vi "SH_ComputeThreshold.vi"(4 "Shapelet Length":i32, 5 "ShapeletClass in":refnum<class "Shapelets Search Brute Force.lvclass">) -> (0 "percentile":dbl, 2 "ShapeletClass out":refnum<class "Shapelets Search Brute Force.lvclass">)   [LabVIEW 2016, in "Shapelets Search (Brute Force).lvlib" / "Shapelets Search Brute Force.lvclass"]
uses:
  Shapelets Search Brute Force.lvclass
  Shapelets Search Brute Force.lvclass/Shapelets Search Brute Force.ctl
  <vilib>/Analysis/baseanly.llb/Normalize Vector.vi
  <vilib>/gmath/statdist.llb/Uniform (Discrete) Random.vi
  <vilib>/gmath/statdist.llb/st_Percentiles (scalar).vi
  <vilib>/gmath/NI_Gmath.lvlib
  <vilib>/Analysis/NI_AALBase.lvlib
panel:
  # "This VI is a part of BCI Design library, http://www.ru-bci.org \nCopyright © 2020, Sotnikov Peter, All rights reserved. License: GNU GPLv3"
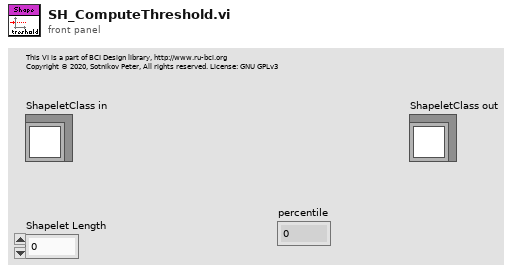
[diagram p1: front panel]
types:
  T1 = cluster{"ClassLabel":string, "FeatureVector":dbl[][]}[]
  T2 = cluster{"ClassLabel":string, "FeatureVector":dbl[][]}
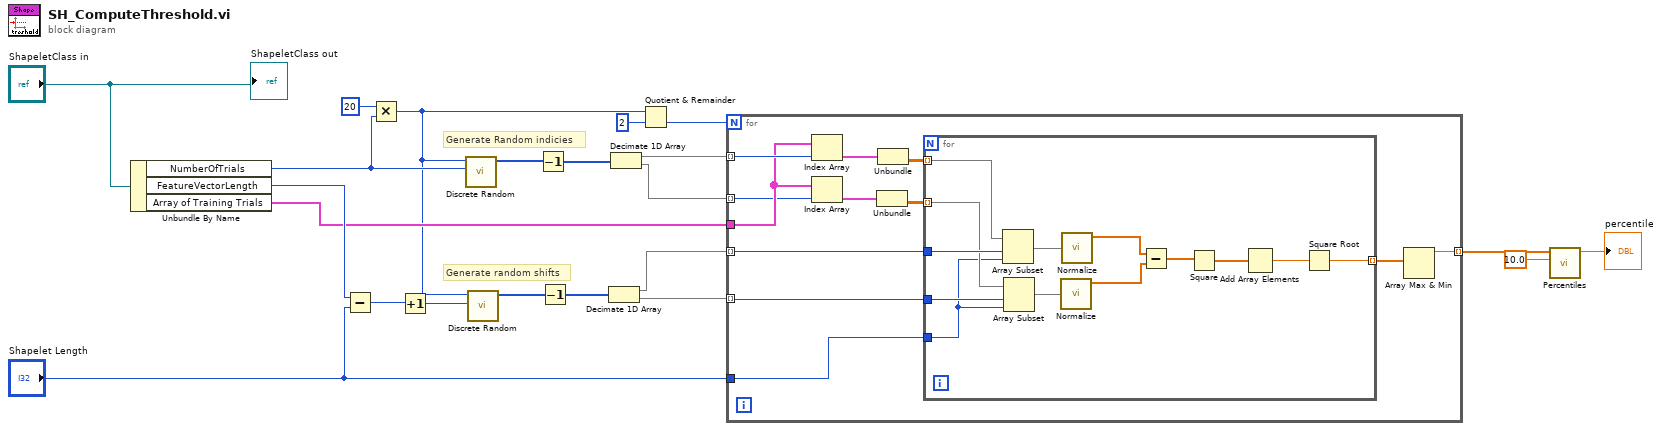
[diagram p0: block diagram]
diagram:
  # "Generate Random indicies"
  # "Generate random shifts"
  n1 = Unbundle By Name("ShapeletClass in") -> ("NumberOfTrials"=w6:i32, "FeatureVectorLength"=w21:i32, "Array of Training Trials"=w14:T1)
  n2 = Subtract(x=w21, y="Shapelet Length") -> (x-y=w8:i32)
  n3 = Multiply(x=20, y=w6) -> (x*y=w5:i32)
  n4 = Increment(x=w8) -> (x+1=w7:i32)
  n5 = call-poly <vilib>:"Discrete Random.vi"("n"=w6, "samples"=w5) -> ("uniform (discrete) random data"=w12:i32[])  [unwired: 8 in, 1 out]
  n6 = call-poly <vilib>:"Discrete Random.vi"("n"=w7, "samples"=w5) -> ("uniform (discrete) random data"=w10:i32[])  [unwired: 8 in, 1 out]
  n7 = Decrement(x=w12) -> (x-1=w11:i32[])
  n8 = Decrement(x=w10) -> (x-1=w9:i32[])
  n9 = Decimate 1D Array(w9) -> (w16:i32[], w15:i32[])
  n10 = Decimate 1D Array(w11) -> (w18:i32[], w17:i32[])
  n11 = Quotient & Remainder(x=w5, y=2) -> (floor(x/y)=w19:i32)  [unwired: 1 out]
  n12 = for {
    N: w19 -> [_]
    tunnel: w18 -> [w34] mode=indexing
    tunnel: w17 -> [w32] mode=indexing
    tunnel: w16 -> [w29] mode=indexing
    tunnel: w15 -> [w28] mode=indexing
    tunnel: w14 -> [w33]
    tunnel: "Shapelet Length" -> [w25]
    tunnel: [w23] -> w3 mode=indexing
    n13 = Index Array(array=w33, index=w34) -> (element=w31:T2)
    n14 = Index Array(array=w33, index=w32) -> (element=w30:T2)
    n15 = Unbundle(w30) -> ("FeatureVector"=w26:dbl[][])  [unwired: 1 out]
    n16 = Unbundle(w31) -> ("FeatureVector"=w27:dbl[][])  [unwired: 1 out]
    n17 = for {
      tunnel: w29 -> [w47]
      tunnel: w28 -> [w46]
      tunnel: w27 -> [w45] mode=indexing
      tunnel: w26 -> [w44] mode=indexing
      tunnel: w25 -> [w37]
      tunnel: [w36] -> w24 mode=indexing
      n18 = Array Subset(array=w45, index=w47, length=w37) -> (w43:dbl[])
      n19 = Array Subset(array=w44, index=w46, length=w37) -> (w42:dbl[])
      n20 = call-poly <vilib>:"Normalize.vi"("Vector"=w42) -> ("Normalized Vector"=w40:dbl[])  [unwired: 1 in, 3 out]
      n21 = call-poly <vilib>:"Normalize.vi"("Vector"=w43) -> ("Normalized Vector"=w41:dbl[])  [unwired: 1 in, 3 out]
      n22 = Subtract(x=w41, y=w40) -> (x-y=w39:dbl[])
      n23 = Square(x=w39) -> (x^2=w38:dbl[])
      n24 = Add Array Elements(numeric array=w38) -> (sum=w35:dbl)
      n25 = Square Root(x=w35) -> (sqrt(x)=w36:dbl)
    }
    n26 = Array Max & Min(array=w24) -> (max value=w23:dbl)  [unwired: 3 out]
  }
  n27 = call-poly <vilib>:"Percentiles.vi"("p"=10.0, "x array"=w3) -> ("percentile"=→"percentile":dbl)  [unwired: 8 in, 1 out]
  "ShapeletClass out" <- "ShapeletClass in"
